vi "MagGainRead.vi"(8 "Error in":errorcluster, 11 "Serial port":refnum<visa-resource-name>="COM28") -> (0 "Error out":errorcluster, 1 "Gain Read":string, 3 "Serial port out":refnum<visa-resource-name>)   [LabVIEW 2012]
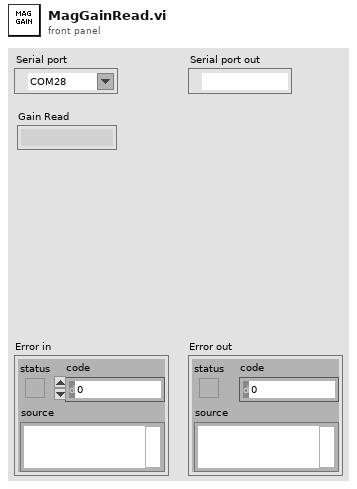
[diagram p1: front panel]
types:
  T1 = enum16{"big-endian, network order", "native, host order", "little-endian"}
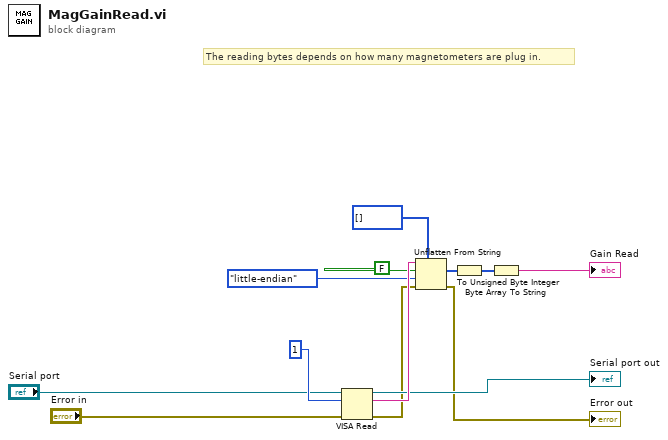
[diagram p0: block diagram]
diagram:
  # "The reading bytes depends on how many magnetometers are plug in."
  n1 = VISA Read(VISA resource name="Serial port", byte count=u32 1, error in (no error)="Error in") -> (VISA resource name out=→"Serial port out":refnum<visa-resource-name>, read buffer=w13:string, error out=w5:errorcluster)  [unwired: 1 out]
  n2 = Unflatten From String(type=i8[] [], binary string=w13, data includes array or string size? (T)=FALSE, byte order (0:big-endian, network order)=T1."little-endian", error in (no error)=w5) -> (value=w3:i8[], error out=→"Error out":errorcluster)  [unwired: 1 out]
  n3 = To Unsigned Byte Integer(number=w3) -> (unsigned 8bit integer=w2:u8[])
  n4 = Byte Array To String(unsigned byte array=w2) -> (string=→"Gain Read":string)
